vi "Mouse Down Discard.vi"(7 "Loopdata.MouseDownState":T1, 8 "PlatMods":T2, 9 "Button":u16, 10 "Coords":T3, 11 "plot reference":refnum<vi>) -> (1 "Discard?":bool, 2 "Start new ToolTip?":bool, 3 "command":T1)   [LabVIEW 2021, in "RocketPlot.lvlib"]
uses:
  RocketPlot.lvlib
  <vilib>/Utility/miscctls.llb/LVPoint32TypeDef.ctl
  TypeDefs/MouseDownState.ctl
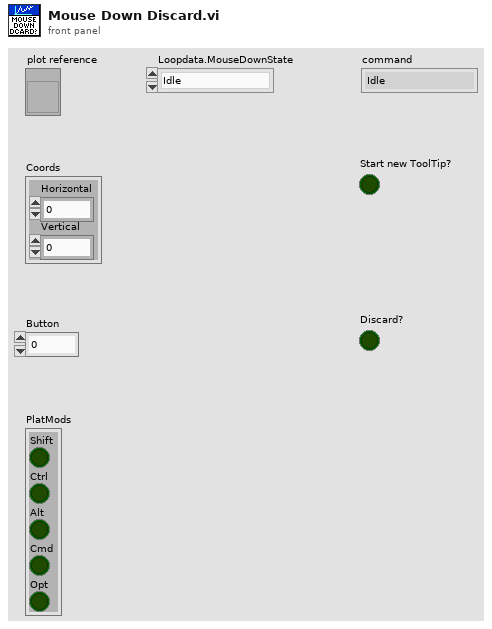
[diagram p1: front panel]
types:
  T1 = typedef "RocketPlot.lvlib/MouseDownState.ctl" = enum16{"Idle", "Pan", "Zoom", "Zoom-Post", "RightClick"}
  T2 = cluster{"Shift":bool, "Ctrl":bool, "Alt":bool, "Cmd":bool, "Opt":bool}
  T3 = typedef "LVPoint32TypeDef.ctl" = cluster{"Horizontal":i32, "Vertical":i32}
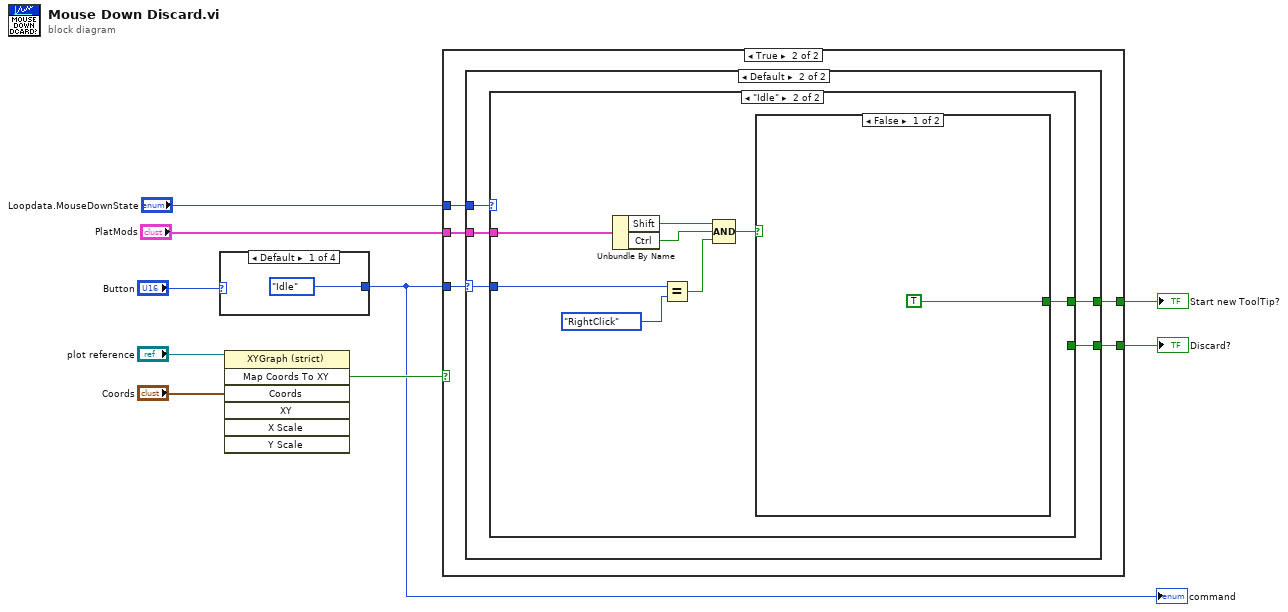
[diagram p0: block diagram]
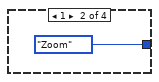
[diagram p2: hidden frame]
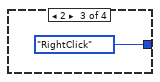
[diagram p3: hidden frame]
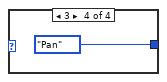
[diagram p4: hidden frame]
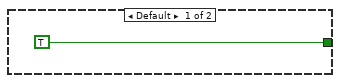
[diagram p7: hidden frame]
diagram:
  n1 = case shown="Default" "Button" {
    tunnel: [MouseDownState."Idle" ("ScaleState") MouseDownState."Zoom" ("ScaleState") MouseDownState."RightClick" ("ScaleState") MouseDownState."Pan" ("ScaleState")] -> w5
    frame Default {
    }
    frame 1 {
    }
    frame 2 {
    }
    frame 3 {
    }
  }
  "command" <- w5
  n2 = invoke class="XYGraph (strict)" method="Map Coords To XY"(reference="plot reference", "Coords"="Coords") -> ("Map Coords To XY"=w6:bool)  [unwired: 5 in, 6 out]
  n3 = case shown="True" w6 {
    tunnel: w5 -> [_ w18]
    tunnel: "Loopdata.MouseDownState" -> [_ w17]
    tunnel: [_ w16] -> w4
    tunnel: [_ w15] -> w3
    tunnel: "PlatMods" -> [_ w14]
    frame False {
    }
    frame True {
      n4 = case shown="Default" w18 {
        selector: w18 -> [_ w19]
        tunnel: w17 -> [_ w23]
        tunnel: [_ w22] -> w16
        tunnel: [_ w21] -> w15
        tunnel: w14 -> [_ w20]
        frame "Idle" {
        }
        frame Default {
          n5 = case shown="\"Idle\"" w23 {
            tunnel: [TRUE _] -> w22
            tunnel: [_ w25] -> w21
            tunnel: w20 -> [_ w30]
            tunnel: w19 -> [_ w32]
            frame Default {
            }
            frame "Idle" {
              n6 = Unbundle By Name(w30) -> ("Shift"=w29:bool, "Ctrl"=w28:bool)
              n7 = Equal?(x=w32, y=MouseDownState."RightClick" ("ScaleState")) -> (x = y?=w27:bool)
              n8 = Compound Arithmetic op=AND(w29, w28, w27) -> (w26:bool)
              n9 = case shown="False" w26 {
                tunnel: [TRUE _] -> w25
                frame False {
                }
                frame True {
                }
              }
            }
          }
        }
      }
    }
  }
  "Discard?" <- w4
  "Start new ToolTip?" <- w3
